vi "Write Error Counts.vi"(8 "error in":errorcluster, 10 "error counts":T1, 11 "Rx execution unit in":refnum<class "Rx Execution Unit.lvclass">) -> (0 "error out":errorcluster, 3 "Rx execution unit out":refnum<class "Rx Execution Unit.lvclass">)   [LabVIEW 2020, in "Ballard ARINC 429 Engine.lvlib" / "Implementation.lvlib" / "Rx Execution Unit.lvclass"]
uses:
  Rx Execution Unit.lvclass
  Rx Execution Unit.lvclass/Rx Execution Unit.ctl
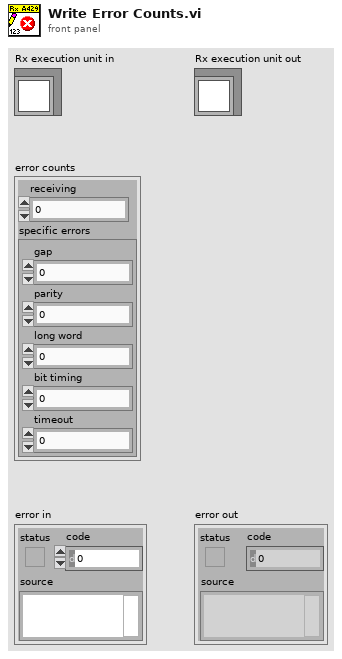
[diagram p1: front panel]
types:
  T1 = cluster{"receiving":dbl, "specific errors":cluster{"gap":dbl, "parity":dbl, "long word ":dbl, "bit timing":dbl, "timeout":dbl}}
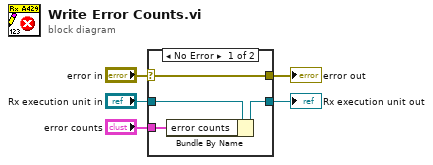
[diagram p0: block diagram]
diagram:
  n1 = case shown="No Error" "error in" {
    selector: "error in" -> [w9 w10]
    tunnel: [w9 w10] -> w4
    tunnel: [w7 w11] -> w2
    tunnel: "Rx execution unit in" -> [w8 w11]
    tunnel: "error counts" -> [w6 _]
    frame No Error {
      n2 = Bundle By Name(cluster=w8, "error counts"=w6) -> (w7:refnum<class "Rx Execution Unit.lvclass">)
    }
    frame Error {
    }
  }
  "error out" <- w4
  "Rx execution unit out" <- w2
